vi "Barrel Race Path.vi"   [LabVIEW 2019]
uses:
  Robot Global Data.vi
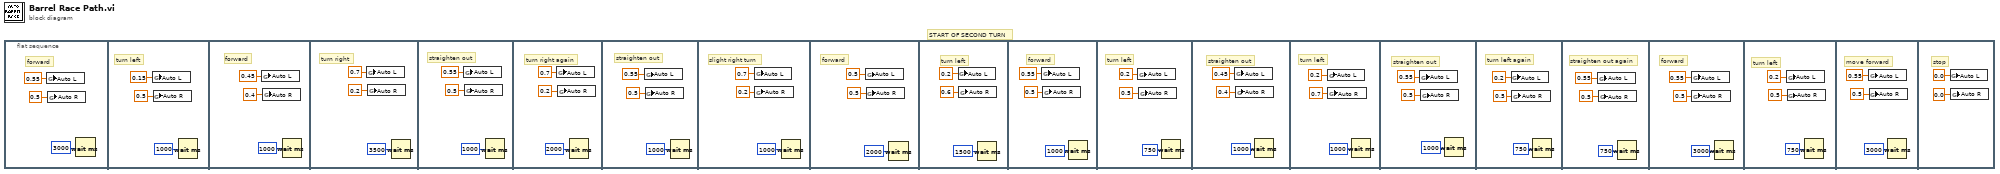
[diagram p0: block diagram]
diagram:
  # "START OF SECOND TURN"
  n1 = flat-sequence {
    frame #0 {
      # "forward"
      n2 = global write "Robot Global Data.vi" "Auto L"(0.55 ("Auto X")) -> ()
      n3 = global write "Robot Global Data.vi" "Auto R"(0.5 ("Auto Y")) -> ()
      n4 = Wait (ms)(milliseconds to wait=u32 3000) -> ()  [unwired: 1 out]
    }
    frame #1 {
      # "turn left"
      n5 = global write "Robot Global Data.vi" "Auto L"(0.15 ("Auto X")) -> ()
      n6 = global write "Robot Global Data.vi" "Auto R"(0.5 ("Auto Y")) -> ()
      n7 = Wait (ms)(milliseconds to wait=u32 1000) -> ()  [unwired: 1 out]
    }
    frame #2 {
      # "forward"
      n8 = global write "Robot Global Data.vi" "Auto L"(0.45 ("Auto X")) -> ()
      n9 = global write "Robot Global Data.vi" "Auto R"(0.4 ("Auto Y")) -> ()
      n10 = Wait (ms)(milliseconds to wait=u32 1000) -> ()  [unwired: 1 out]
    }
    frame #3 {
      # "turn right"
      n11 = global write "Robot Global Data.vi" "Auto L"(0.7 ("Auto X")) -> ()
      n12 = global write "Robot Global Data.vi" "Auto R"(0.2 ("Auto Y")) -> ()
      n13 = Wait (ms)(milliseconds to wait=u32 3500) -> ()  [unwired: 1 out]
    }
    frame #4 {
      # "straighten out"
      n14 = global write "Robot Global Data.vi" "Auto L"(0.55 ("Auto X")) -> ()
      n15 = global write "Robot Global Data.vi" "Auto R"(0.5 ("Auto Y")) -> ()
      n16 = Wait (ms)(milliseconds to wait=u32 1000) -> ()  [unwired: 1 out]
    }
    frame #5 {
      # "turn right again"
      n17 = global write "Robot Global Data.vi" "Auto L"(0.7 ("Auto X")) -> ()
      n18 = global write "Robot Global Data.vi" "Auto R"(0.2 ("Auto Y")) -> ()
      n19 = Wait (ms)(milliseconds to wait=u32 2000) -> ()  [unwired: 1 out]
    }
    frame #6 {
      # "straighten out"
      n20 = global write "Robot Global Data.vi" "Auto L"(0.55 ("Auto X")) -> ()
      n21 = global write "Robot Global Data.vi" "Auto R"(0.5 ("Auto Y")) -> ()
      n22 = Wait (ms)(milliseconds to wait=u32 1000) -> ()  [unwired: 1 out]
    }
    frame #7 {
      # "slight right turn"
      n23 = global write "Robot Global Data.vi" "Auto L"(0.7 ("Auto X")) -> ()
      n24 = global write "Robot Global Data.vi" "Auto R"(0.2 ("Auto Y")) -> ()
      n25 = Wait (ms)(milliseconds to wait=u32 1000) -> ()  [unwired: 1 out]
    }
    frame #8 {
      # "forward"
      n26 = global write "Robot Global Data.vi" "Auto L"(0.5 ("Auto X")) -> ()
      n27 = global write "Robot Global Data.vi" "Auto R"(0.5 ("Auto Y")) -> ()
      n28 = Wait (ms)(milliseconds to wait=u32 2000) -> ()  [unwired: 1 out]
    }
    frame #9 {
      # "turn left"
      n29 = global write "Robot Global Data.vi" "Auto L"(0.2 ("Auto X")) -> ()
      n30 = global write "Robot Global Data.vi" "Auto R"(0.6 ("Auto Y")) -> ()
      n31 = Wait (ms)(milliseconds to wait=u32 1500) -> ()  [unwired: 1 out]
    }
    frame #10 {
      # "forward"
      n32 = global write "Robot Global Data.vi" "Auto L"(0.55 ("Auto X")) -> ()
      n33 = global write "Robot Global Data.vi" "Auto R"(0.5 ("Auto Y")) -> ()
      n34 = Wait (ms)(milliseconds to wait=u32 1000) -> ()  [unwired: 1 out]
    }
    frame #11 {
      # "turn left"
      n35 = global write "Robot Global Data.vi" "Auto L"(0.2 ("Auto X")) -> ()
      n36 = global write "Robot Global Data.vi" "Auto R"(0.5 ("Auto Y")) -> ()
      n37 = Wait (ms)(milliseconds to wait=u32 750) -> ()  [unwired: 1 out]
    }
    frame #12 {
      # "straighten out"
      n38 = global write "Robot Global Data.vi" "Auto L"(0.45 ("Auto X")) -> ()
      n39 = global write "Robot Global Data.vi" "Auto R"(0.4 ("Auto Y")) -> ()
      n40 = Wait (ms)(milliseconds to wait=u32 1000) -> ()  [unwired: 1 out]
    }
    frame #13 {
      # "turn left"
      n41 = global write "Robot Global Data.vi" "Auto L"(0.2 ("Auto X")) -> ()
      n42 = global write "Robot Global Data.vi" "Auto R"(0.7 ("Auto Y")) -> ()
      n43 = Wait (ms)(milliseconds to wait=u32 1000) -> ()  [unwired: 1 out]
    }
    frame #14 {
      # "straighten out"
      n44 = global write "Robot Global Data.vi" "Auto L"(0.55 ("Auto X")) -> ()
      n45 = global write "Robot Global Data.vi" "Auto R"(0.5 ("Auto Y")) -> ()
      n46 = Wait (ms)(milliseconds to wait=u32 1000) -> ()  [unwired: 1 out]
    }
    frame #15 {
      # "turn left again"
      n47 = global write "Robot Global Data.vi" "Auto L"(0.2 ("Auto X")) -> ()
      n48 = global write "Robot Global Data.vi" "Auto R"(0.5 ("Auto Y")) -> ()
      n49 = Wait (ms)(milliseconds to wait=u32 750) -> ()  [unwired: 1 out]
    }
    frame #16 {
      # "straighten out again"
      n50 = global write "Robot Global Data.vi" "Auto L"(0.55 ("Auto X")) -> ()
      n51 = global write "Robot Global Data.vi" "Auto R"(0.5 ("Auto Y")) -> ()
      n52 = Wait (ms)(milliseconds to wait=u32 750) -> ()  [unwired: 1 out]
    }
    frame #17 {
      # "forward"
      n53 = global write "Robot Global Data.vi" "Auto L"(0.55 ("Auto X")) -> ()
      n54 = global write "Robot Global Data.vi" "Auto R"(0.5 ("Auto Y")) -> ()
      n55 = Wait (ms)(milliseconds to wait=u32 3000) -> ()  [unwired: 1 out]
    }
    frame #18 {
      # "turn left"
      n56 = global write "Robot Global Data.vi" "Auto L"(0.2 ("Auto X")) -> ()
      n57 = global write "Robot Global Data.vi" "Auto R"(0.5 ("Auto Y")) -> ()
      n58 = Wait (ms)(milliseconds to wait=u32 750) -> ()  [unwired: 1 out]
    }
    frame #19 {
      # "move forward"
      n59 = global write "Robot Global Data.vi" "Auto L"(0.55 ("Auto X")) -> ()
      n60 = global write "Robot Global Data.vi" "Auto R"(0.5 ("Auto Y")) -> ()
      n61 = Wait (ms)(milliseconds to wait=u32 3000) -> ()  [unwired: 1 out]
    }
    frame #20 {
      # "stop"
      n62 = global write "Robot Global Data.vi" "Auto L"(0.0 ("Auto X")) -> ()
      n63 = global write "Robot Global Data.vi" "Auto R"(0.0 ("Auto Y")) -> ()
    }
  }
